vi "send&receive_img.vi"() -> ()   [LabVIEW 2018, in "LV-Julia_ZMQ-Roundtrip_lib.lvlib"]
uses:
  LV-Julia_ZMQ-Roundtrip_lib.lvlib
  Server or client state.ctl
  detailed error info.ctl
  StackFrame.ctl
  Bindata description.ctl
  <vilib>/picture/picture.llb/imagedata.ctl
  Commands v2.ctl
  commands LV2Jl.ctl
  d2cb43a9-9305-42fb-ad58-bce983510195.vi
  d2cb43a9-9305-42fb-ad58-bce983510195.vi/de9e5448-4b5f-441e-8b3f-77a70dbcf496.vi
  d2cb43a9-9305-42fb-ad58-bce983510195.vi/7a2aeb1d-c379-4d90-aa08-4860683a5f18.vi
  d2cb43a9-9305-42fb-ad58-bce983510195.vi/611d9bbb-6efa-4863-9150-13229085b8ee.vi
  check ID validity.vi
  bindata_descr to JSON.vi
  check cluster field names.vi
  concat JSON.vi
panel:
  out "images":bool
  out "x = y?":bool
  out "image sent":T1
  out "img received":T1
  out "Bindata & descr out":cluster{"bindata_descr":T2[], "bindata":u8[]}
  out "size received":i32
  out "size sent":i32
  out "bindata":u8[](array[numeric])
  out "flattened data out":u8[](array[numeric])
  out "picture dup":picture
  in  "peppers":bool
  in  "Path":path=path "C:/_MyOwnDocs/MyTmp/ScreenShots/2019-07-30 14_38_29-Desktop Execution Trace Toolkit.png"
  out "picture":picture
  in  "next":bool
  in  "stop LV only":bool
  in  "stop":bool
  out "detailed error info":T3
  in  "params":cluster{"idx":u16[], "showversion":bool}={"idx"=[3000, 4000], "showversion"=TRUE} {"idx" min=1}
  out "Jl Server state out":T5
  out "short err code":u8
  out "final error":errorcluster
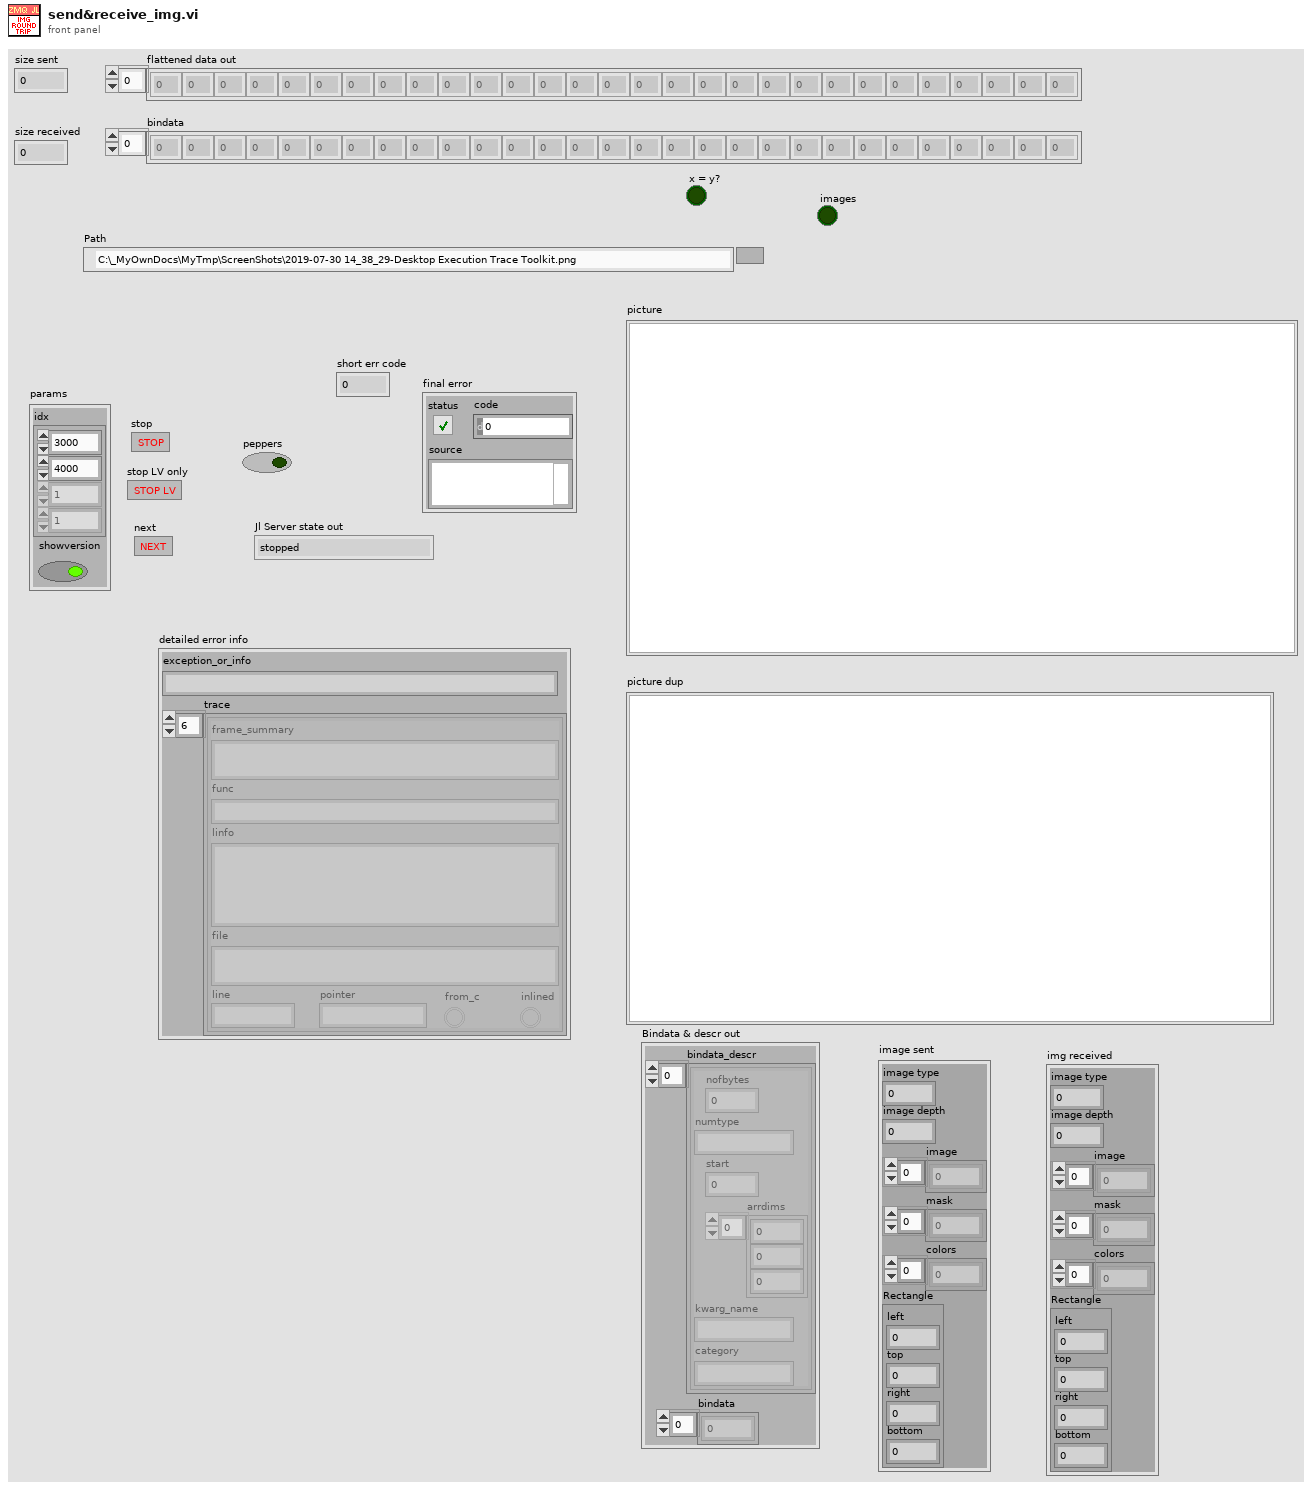
[diagram p1: front panel]
types:
  T1 = typedef "imagedata.ctl" = cluster{"image type":i32, "image depth":i32, "image":u8[], "mask":u8[], "colors":u32[], "Rectangle":cluster{"left":i16, "top":i16, "right":i16, "bottom":i16}}
  T2 = typedef "LV-Julia_ZMQ-Roundtrip_lib.lvlib/Bindata description.ctl" = cluster{"nofbytes":i32, "numtype":string, "start":i32, "arrdims":i32[], "kwarg_name":string, "category":string}
  T3 = typedef "LV-Julia_ZMQ-Roundtrip_lib.lvlib/detailed error info.ctl" = cluster{"exception_or_info":string, "trace":T4[]}
  T4 = typedef "LV-Julia_ZMQ-Roundtrip_lib.lvlib/StackFrame.ctl" = cluster{"frame_summary":string, "func":string, "linfo":string, "file":string, "line":i32, "pointer":u64, "from_c":bool, "inlined":bool}
  T5 = typedef "LV-Julia_ZMQ-Roundtrip_lib.lvlib/Server or client state.ctl" = enum16{"stopped", "running", "unknown"}
  T6 = typedef "LV-Julia_ZMQ-Roundtrip_lib.lvlib/Commands v2.ctl" = enum16{"Start Jl-server & Init LV-client", "Send request & Get response ", "Stop Jl-server & Cleanup LV-client", "Cleanup LV-client", "Start Jl-server", "Stop Jl-server", "Init LV-Client", "Cleanup LV-Client", "(not allowed)", "Set LV Client state", "Set Jl Server state"}
  T7 = typedef "commands LV2Jl.ctl" = u8
  T8 = typedef "Bindata&description.ctl" = cluster{"bindata_descr":T2[], "bindata":u8[]}
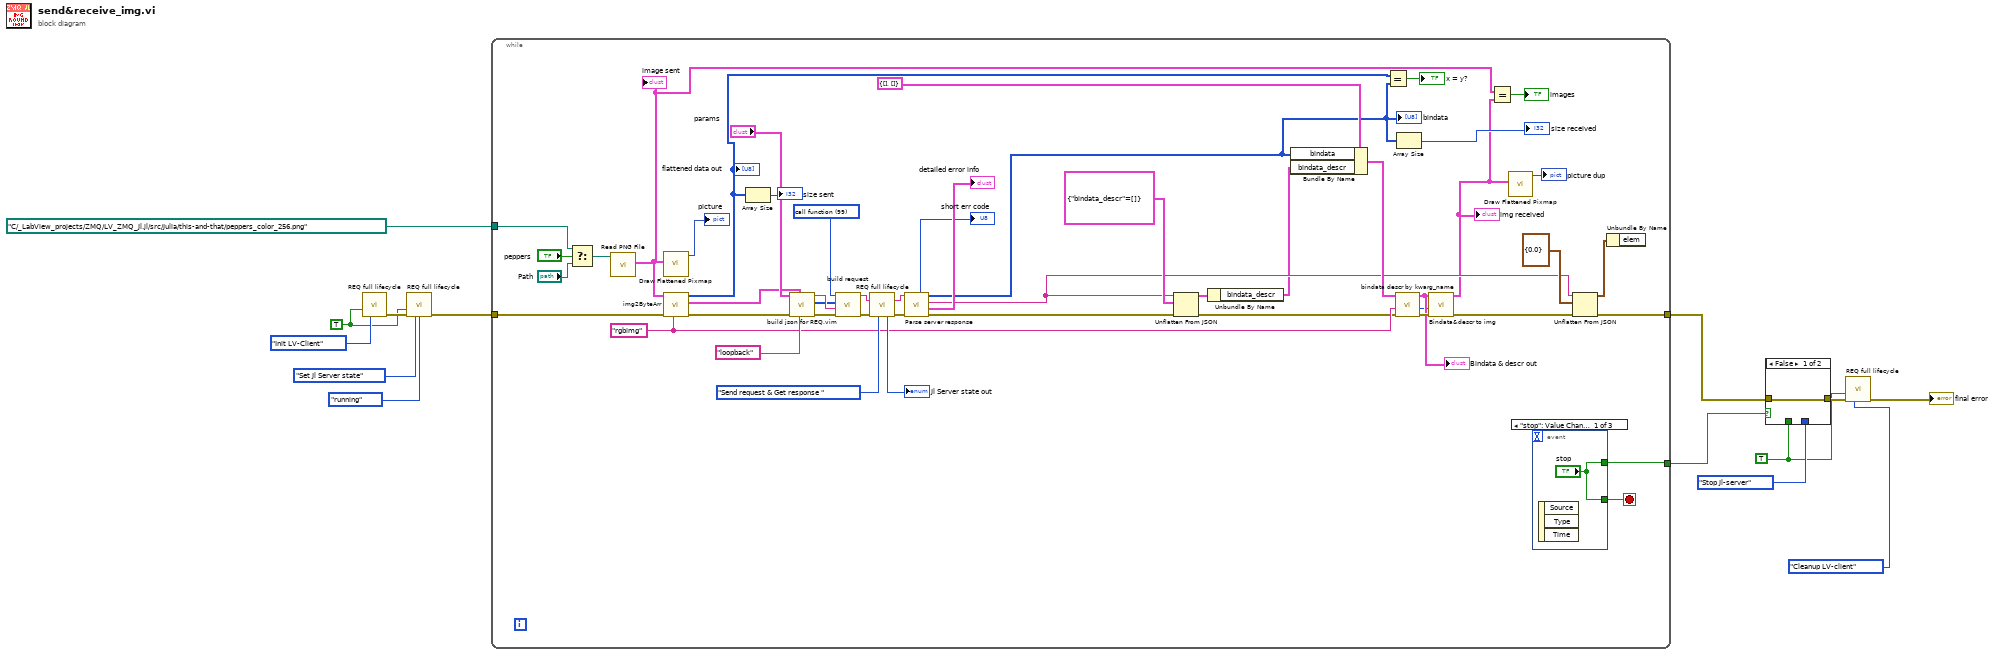
[diagram p0: block diagram]
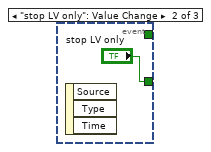
[diagram p2: hidden frame]
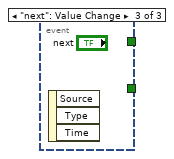
[diagram p3: hidden frame]
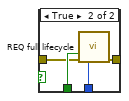
[diagram p4: hidden frame]
diagram:
  w6 = TRUE ("Force command")
  w10 = TRUE ("Force command")
  n1 = call "REQ full lifecycle.vi"("Force command"=w6, "command"=Commands_v2."Init LV-Client") -> ("error out"=w8:errorcluster)  [unwired: 10 in, 3 out]
  n2 = call "REQ full lifecycle.vi"("Force command"=w6, "error in"=w8, "command"=Commands_v2."Set Jl Server state", "Jl Server state in"=Server_or_client_state."running") -> ("error out"=w4:errorcluster)  [unwired: 8 in, 3 out]
  n3 = while {
    tunnel: w4 -> [w39]
    tunnel: [w49] -> w3
    tunnel: path "C:/_LabView_projects/ZMQ/LV_ZMQ_Jl.jl/src/Julia/this-and-that/peppers_color_256.png" ("Path") -> [w41]
    tunnel: [w37] -> w1
    stop <- w50 stop-if-true
    w32 = "rgbimg" ("Tag")
    w57 = T7 99 items=["call function"=99, "ping"=112, "stop"=115] ("Command")
    n4 = Select(t=w41, s="peppers", f="Path") -> (s? t:f=w42:path)
    n5 = call <vilib>:"Read PNG File.vi"("path to PNG file"=w42) -> ("image data"=w15:T1)  [unwired: 8 in, 2 out]
    "image sent" <- w15
    n6 = call <vilib>:"Draw Flattened Pixmap.vi"("image data"=w15) -> ("new picture"=→"picture":picture)  [unwired: 8 in]
    n7 = call "img2ByteArr.vi"("kwarg_name"=w32, "error in (no error)"=w39, "img in"=w15) -> ("error out"=w40:errorcluster, "Bindata & descr out"=w38:T8, "flattened data out"=w19:u8[])  [unwired: 6 in]
    "flattened data out" <- w19
    n8 = Array Size(array=w19) -> (size(s)=→"size sent":i32)
    n9 = call "build json for REQ.vim"("fun2call"="loopback", "Bindata & descr in"=w38, "error in (no error)"=w40, "Arguments 1"="params") -> ("error out"=w62:errorcluster, "bindata out"=w52:u8[], "JSON string out"=w53:string)  [unwired: 5 in]
    n10 = call "build request.vi"("error in (no error)"=w62, "JSON data"=w53, "binary data"=w52, "Command"=w57) -> ("error out"=w60:errorcluster, "REQ string"=w61:string)  [unwired: 6 in]
    n11 = call "REQ full lifecycle.vi"("data to send"=w61, "error in"=w60, "command"=Commands_v2."Send request & Get response ") -> ("server response"=w55:string, "Jl Server state out"=→"Jl Server state out":T5, "error out"=w59:errorcluster)  [unwired: 9 in, 1 out]
    n12 = call "Parse server response.vi"("error in (no error)"=w59, "server response in"=w55) -> ("error out"=w26:errorcluster, "detailed error info"=→"detailed error info":T3, "JSON out"=w27:string, "binary data"=w20:u8[], "return code"=→"short err code":u8)  [unwired: 3 in, 2 out]
    "bindata" <- w20
    n13 = Unflatten From JSON(JSON string=w27, type and defaults=cluster{"bindata_descr":T2[]} {"bindata_descr"=[]}, error in (no error)=w26) -> (value=w28:cluster{"bindata_descr":T2[]}, error out=w23:errorcluster)  [unwired: 4 in]
    n14 = Unbundle By Name(w28) -> ("bindata_descr"=w25:T2[])
    n15 = Bundle By Name(cluster=cluster{"bindata_descr":T2[], "bindata":u8[]} {"bindata_descr"=[], "bindata"=[]} ("Bindata & descr"), "bindata"=w20, "bindata_descr"=w25) -> (w30:cluster{"bindata_descr":T2[], "bindata":u8[]})
    n16 = Equal?(x=w19, y=w20) -> (x = y?=→"x = y?":bool)
    n17 = call "bindata descr by kwarg_name.vi"("Error in"=w23, "kwarg_name"=w32, "Bindata & descr"=w30) -> ("Error out"=w35:errorcluster, "index"=w33:i32, "Bindata & descr out"=w34:cluster{"bindata_descr":T2[], "bindata":u8[]})  [unwired: 5 in, 1 out]
    "Bindata & descr out" <- w34
    n18 = Array Size(array=w20) -> (size(s)=→"size received":i32)
    n19 = call "Bindata&descr to img.vi"("error in (no error)"=w35, "bindata_descr index"=w33, "Bindata & descr in"=w34) -> ("error out"=w24:errorcluster, "img out"=w16:T1)  [unwired: 7 in]
    "img received" <- w16
    n20 = Equal?(x=w15, y=w16) -> (x = y?=→"images":bool)
    n21 = call <vilib>:"Draw Flattened Pixmap.vi"("image data"=w16) -> ("new picture"=→"picture dup":picture)  [unwired: 8 in]
    n22 = event shown="[0] \"stop\": Value Change" {
      selector: _ -> [_ _ _]
      dyn-events: _ -> [_ _ _]
      timeout: _ -> [_ _ _]
      tunnel: ["stop" "stop LV only" _] -> w50
      tunnel: ["stop" _ _] -> w49
      event "stop": Value Change {
        n23 = event-data() -> ()  [unwired: 1 in, 3 out]
      }
      event "stop LV only": Value Change {
        n24 = event-data() -> ()  [unwired: 1 in, 3 out]
      }
      event "next": Value Change {
        n25 = event-data() -> ()  [unwired: 1 in, 3 out]
      }
    }
    n26 = Unflatten From JSON(JSON string=w27, type and defaults=cluster{"elem":dbl} {"elem"=0.0} ("parsed response"), error in (no error)=w24) -> (value=w47:cluster{"elem":dbl}, error out=w37:errorcluster)  [unwired: 4 in]
    n27 = Unbundle By Name(w47) -> ()  [unwired: 1 out]
  }
  n28 = case shown="False" w3 {
    tunnel: Commands_v2."Stop Jl-server" ("command") -> [_ w70]
    tunnel: [w66 w69] -> w13
    tunnel: w10 -> [_ w68]
    tunnel: w1 -> [w66 w67]
    frame False {
    }
    frame True {
      n29 = call "REQ full lifecycle.vi"("Force command"=w68, "error in"=w67, "command"=w70) -> ("error out"=w69:errorcluster)  [unwired: 9 in, 3 out]
    }
  }
  n30 = call "REQ full lifecycle.vi"("Force command"=w10, "error in"=w13, "command"=Commands_v2."Cleanup LV-client") -> ("error out"=→"final error":errorcluster)  [unwired: 9 in, 3 out]
